vi "Autofocus.vi"(0 "controller in":refnum<k24>, 1 "AbortAutoFocus":bool, 5 "SafeMaxZ":dbl=86.0 format="%#_13g", 7 "InitialStepSize":dbl=0.1, 9 "Tolerance":dbl=0.005 format="%#_13g", 11 "error in (no error)":errorcluster) -> (4 "controller out":refnum<k24>, 6 "Image":T2(plugin-control), 8 "N_iterations":dbl, 10 "BestZvalue":dbl, 15 "error out":errorcluster)   [LabVIEW 2019]
uses:
  C:/Users/TTUHEP/Documents/LabVIEW/Other Models/2010/Bin/Aerotech.A3200.dll
  Other Models/2010/Bin/Aerotech.A3200.dll
  <vilib>/userDefined/High Color/IMAQdx.ctl
  <vilib>/vision/NI_Vision_Development_Module.lvlib
  <vilib>/vision/driver/NI_Vision_Acquisition_Software.lvlib
panel:
  out "ZvsSD":string
  in  "Camera":T1="cam1"
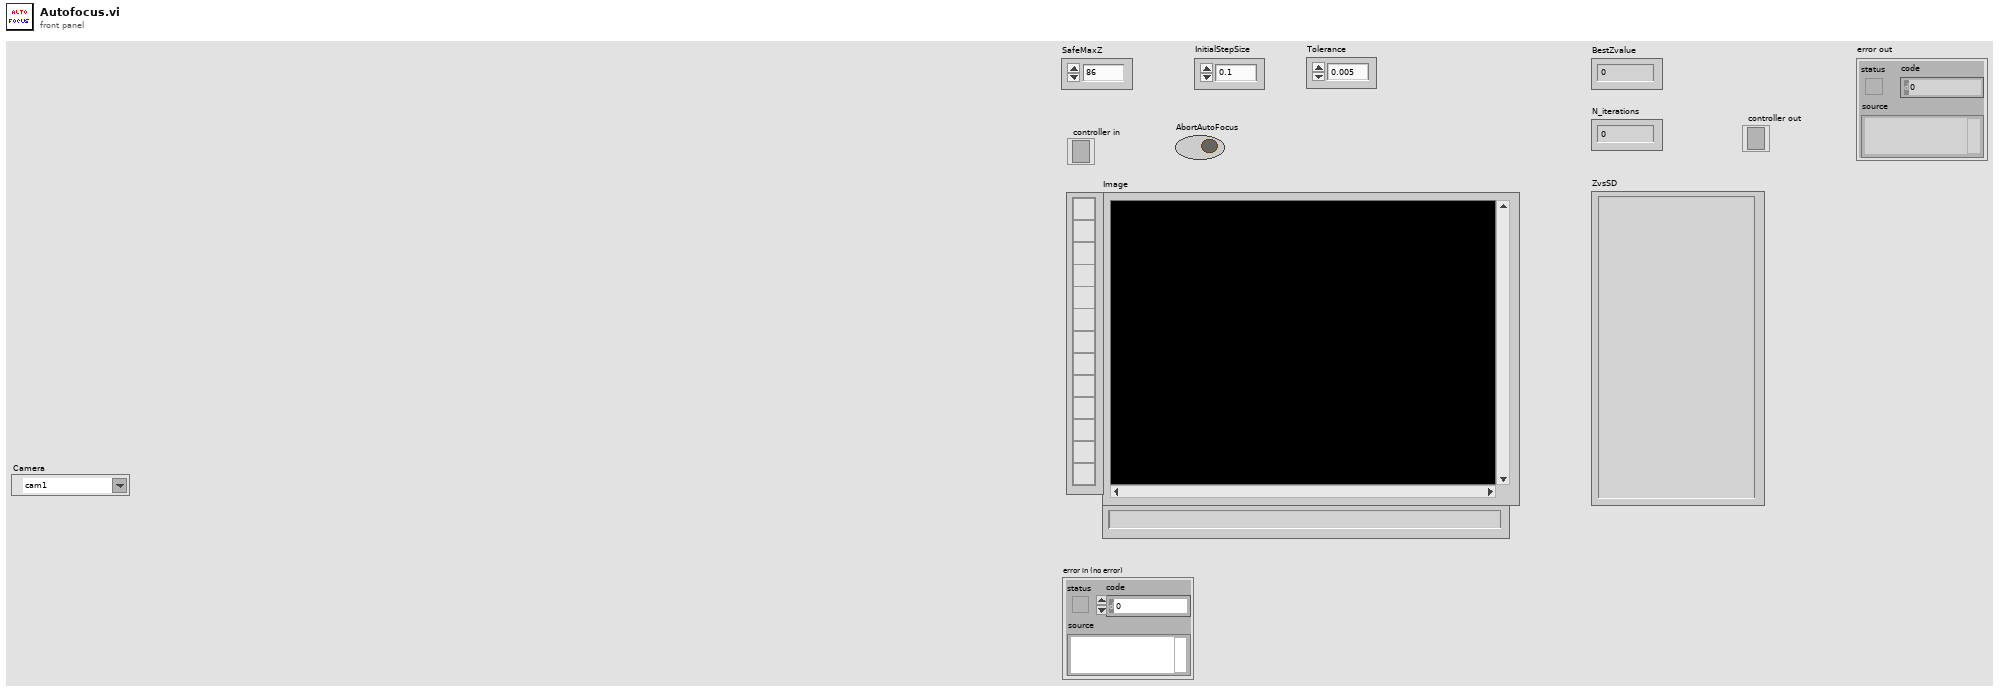
[diagram p1: front panel]
types:
  T1 = typedef "IMAQdx.ctl" = refnum<k21>
  T2 = typedef "IMAQ Image.ctl" = refnum<image>
  T3 = typedef "Image Type" = u32
  T4 = enum32{"Differentiation", "Gradient", "Prewitt", "Roberts", "Sigma", "Sobel"}
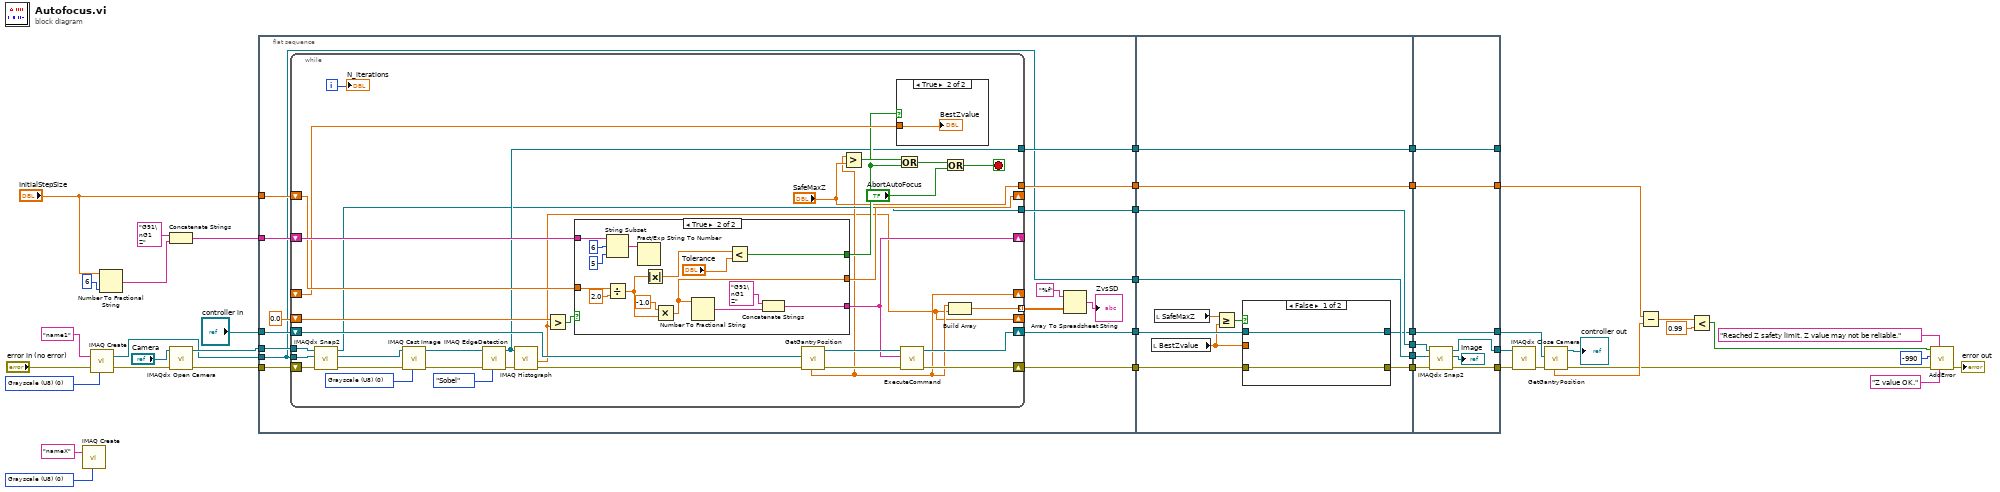
[diagram p0: block diagram]
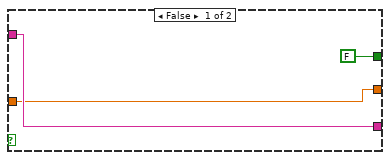
[diagram p3: hidden frame]
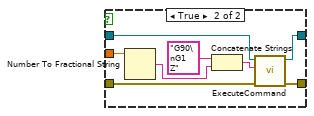
[diagram p4: hidden frame]
diagram:
  w14 = T3 0 items=["Grayscale (U8)", "Grayscale (I16)", "Grayscale (SGL)", "Complex (CSG)", "RGB (U32)", "HSL (U32)", "RGB (U64)", "Grayscale (U16)"] ("Image Type")
  w19 = T3 0 items=["Grayscale (U8)", "Grayscale (I16)", "Grayscale (SGL)", "Complex (CSG)", "RGB (U32)", "HSL (U32)", "RGB (U64)", "Grayscale (U16)"] ("Image Type")
  n1 = call "IMAQ Create"("Image Name"="nameX", "Image Type"=w14) -> ()  [unwired: 3 in, 2 out]
  n2 = call "IMAQ Create"("Image Name"="name1" ("ImageName"), "Image Type"=w19, "error in (no error)"="error in (no error)") -> ("New Image"=w16:T2, "error out"=w21:errorcluster)  [unwired: 2 in]
  n3 = Number To Fractional String(number="InitialStepSize", precision (6)=i16 6) -> (F-format string=w38:string)  [unwired: 2 in]
  n4 = Concatenate Strings("G91\nG1 Z", w38) -> (w40:string)
  n5 = call <vilib>:"IMAQdx Open Camera.vi"("error in"=w21, "Session In"="Camera") -> ("error out"=w18:errorcluster, "Session Out"=w17:T1)  [unwired: 8 in]
  n6 = flat-sequence {
    tunnel: "controller in" -> [w58]
    tunnel: "InitialStepSize" -> [w56]
    tunnel: w40 -> [w55]
    tunnel: w18 -> [w54]
    tunnel: [w53] -> w12
    tunnel: [w52] -> w10
    tunnel: [w51] -> w8
    tunnel: [w50] -> w6
    tunnel: [w48] -> w4
    tunnel: w17 -> [w49]
    tunnel: w16 -> [w47]
    tunnel: [w47] -> w2
    tunnel: w12 -> [w119]
    tunnel: [w116] -> w11
    tunnel: w10 -> [w123]
    tunnel: [w123] -> w9
    tunnel: w8 -> [w118]
    tunnel: [w117] -> w7
    tunnel: w6 -> [w122]
    tunnel: [w122] -> w5
    tunnel: w4 -> [w121]
    tunnel: [w121] -> w3
    tunnel: w2 -> [w120]
    tunnel: [w120] -> w1
    tunnel: [w140] -> _
    tunnel: [w141] -> w25
    tunnel: [w142] -> w37
    tunnel: w11 -> [w142]
    tunnel: w9 -> [w141]
    tunnel: w7 -> [w139]
    tunnel: w5 -> [w140]
    tunnel: [w138] -> w24
    tunnel: [w137] -> w23
    tunnel: w3 -> [w135]
    tunnel: w1 -> [w134]
    frame #0 {
      n7 = while {
        shift-right: [w85] -> w53
        shift-left: w58 -> [w89]
        shift-right: [w87] -> w51
        shift-left: w54 -> [w68]
        shift-right: [w82] -> _
        shift-left: w55 -> [w81]
        shift-right: [w59] -> _
        shift-left: 0.0 -> [w84]
        shift-right: [w78] -> _
        shift-left: w56 -> [w77]
        shift-right: [w60] -> _
        shift-left: _ -> [w76]
        tunnel: ["SafeMaxZ"] -> w52
        tunnel: [w70] -> w50
        tunnel: w47 -> [w66]
        tunnel: w49 -> [w67]
        tunnel: [w64] -> w48
        tunnel: [w61] -> w44 mode=indexing
        i -> [w73]
        stop <- w91 stop-if-true
        w74 = T3 0 items=["Grayscale (U8)", "Grayscale (I16)", "Grayscale (SGL)", "Complex (CSG)", "RGB (U32)", "HSL (U32)", "RGB (U64)", "Grayscale (U16)"] ("Image Type")
        n8 = call <vilib>:"IMAQdx Snap2.vi"("error in"=w68, "Image In"=w66, "Session In"=w67) -> ("error out"=w69:errorcluster, "Image Out"=w65:T2, "Session Out"=w64:T1)  [unwired: 6 in]
        n9 = call "IMAQ Cast Image"("Image Type"=w74, "error in (no error)"=w69, "Image Src"=w65) -> ("error out"=w62:errorcluster, "Image Dst Out"=w90:T2)  [unwired: 7 in]
        n10 = call "IMAQ EdgeDetection"("Method"=T4."Sobel", "error in (no error)"=w62, "Image Src"=w90) -> ("error out"=w93:errorcluster, "Image Dst Out"=w70:T2)  [unwired: 7 in]
        n11 = call "IMAQ Histograph"("error in (no error)"=w93, "Image"=w70) -> ("error out"=w71:errorcluster, "Standard  Deviation"=w59:sgl)  [unwired: 6 in, 2 out]
        n12 = Greater?(x=w84, y=w59) -> (0:w83:bool)
        n13 = case shown="True" w83 {
          tunnel: [w97 w111] -> w82
          tunnel: w81 -> [w97 w105]
          tunnel: [FALSE w106] -> w75
          tunnel: [w95 w101] -> w78
          tunnel: w77 -> [w95 w100]
          frame False {
          }
          frame True {
            n14 = String Subset(string=w105, offset (0)=6, length (rest)=5) -> (substring=w102:string)
            n15 = Divide(x=w100, y=2.0) -> (x/y=w99:dbl)
            n16 = Fract/Exp String To Number(string=w102) -> ()  [unwired: 3 in, 2 out]
            n17 = Absolute Value(x=w99) -> (abs(x)=w98:dbl)
            n18 = Multiply(x=-1.0, y=w99) -> (x*y=w101:dbl)
            n19 = Number To Fractional String(number=w101) -> (F-format string=w110:string)  [unwired: 3 in]
            n20 = Less?(x=w98, y="Tolerance") -> (x < y?=w106:bool)
            n21 = Concatenate Strings("G91\nG1 Z", w110) -> (w111:string)
          }
        }
        n22 = call "GetGantryPosition.vi"("error in (no error)"=w71, "Controller In"=w89) -> ("error out"=w88:errorcluster, "controller out"=w86:refnum<k24>, "Position Z"=w60:dbl)  [unwired: 3 in, 4 out]
        n23 = Greater?(x=w60, y="SafeMaxZ") -> (0:w80:bool)
        n24 = case shown="True" w75 {
          tunnel: w76 -> [_ w94]
          frame False {
          }
          frame True {
            "BestZvalue" <- w94
          }
        }
        n25 = Or(x=w80, y=w75) -> (x .or. y?=w79:bool)
        n26 = call "ExecuteCommand.vi"("error in (no error)"=w88, "Command Code"=w82, "controller in"=w86) -> ("error out"=w87:errorcluster, "controller out"=w85:refnum<k24>)  [unwired: 6 in, 1 out]
        n27 = Or(x=w79, y="AbortAutoFocus") -> (x .or. y?=w91:bool)
        n28 = Build Array(w60, w59) -> (w61:dbl[])
        "N_iterations" <- w73
      }
      n29 = Array To Spreadsheet String(array=w44, 3:"%f" ("format string")) -> (spreadsheet string=→"ZvsSD":string)  [unwired: 1 in]
    }
    frame #1 {
      n30 = local read "BestZvalue"() -> (w114:dbl)
      n31 = local read "SafeMaxZ"() -> (w115:dbl)
      n32 = Greater Or Equal?(x=w115, y=w114) -> (x >= y?=w113:bool)
      n33 = case shown="False" w113 {
        tunnel: w119 -> [w125 w133]
        tunnel: w118 -> [w124 w132]
        tunnel: [w124 w128] -> w117
        tunnel: [w125 w127] -> w116
        tunnel: w114 -> [_ w126]
        frame False {
        }
        frame True {
          n34 = Number To Fractional String(number=w126) -> (F-format string=w131:string)  [unwired: 3 in]
          n35 = Concatenate Strings("G90\nG1 Z", w131) -> (w129:string)
          n36 = call "ExecuteCommand.vi"("error in (no error)"=w132, "Command Code"=w129, "controller in"=w133) -> ("error out"=w128:errorcluster, "controller out"=w127:refnum<k24>)  [unwired: 6 in, 1 out]
        }
      }
    }
    frame #2 {
      n37 = call <vilib>:"IMAQdx Snap2.vi"("error in"=w139, "Image In"=w134, "Session In"=w135) -> ("error out"=w138:errorcluster, "Image Out"=→"Image":T2, "Session Out"=w137:T1)  [unwired: 6 in]
    }
  }
  n38 = call <vilib>:"IMAQdx Close Camera.vi"("error in"=w24, "Session In"=w23) -> ("error out"=w36:errorcluster)  [unwired: 9 in]
  n39 = call "GetGantryPosition.vi"("error in (no error)"=w36, "Controller In"=w37) -> ("error out"=w29:errorcluster, "controller out"=→"controller out":refnum<k24>, "Position Z"=w34:dbl)  [unwired: 3 in, 4 out]
  n40 = Subtract(x=w25, y=w34) -> (x-y=w33:dbl)
  n41 = Less?(x=w33, y=0.99) -> (x < y?=w31:bool)
  n42 = call "AddError.vi"("NoErrorMessage"="Z value OK.", "ErrorMessage"="Reached Z safety limit. Z value may not be reliable.", "error in"=w29, "code"=-990, "Error?"=w31) -> ("Error out"=→"error out":errorcluster)  [unwired: 6 in]
